vi "TestXYGraph_Buffer_Dbl_VIG.vi"(7 "Operation":T1(ring)=enum."set data", 8 "error in":errorcluster, 9 "XYCluster":cluster{"X":dbl, "Y":dbl}, 10 "index/size":i32, 11 "XY_data_in":cluster{"X":dbl, "Y":dbl}[](array[cluster])) -> (0 "error out":errorcluster, 3 "XY_data_out":cluster{"X":dbl, "Y":dbl}[](array[cluster]))   [LabVIEW 2018]
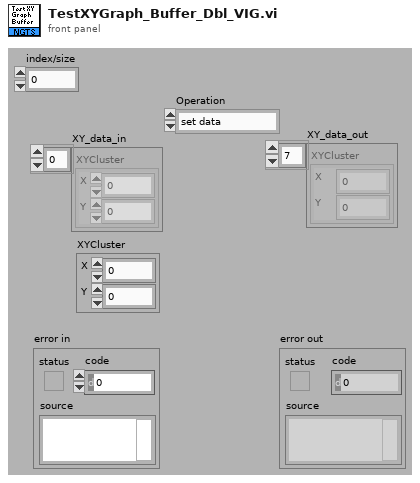
[diagram p1: front panel]
types:
  T1 = enum16{"get data", "set data", "Add Data Pair", "initialize"}
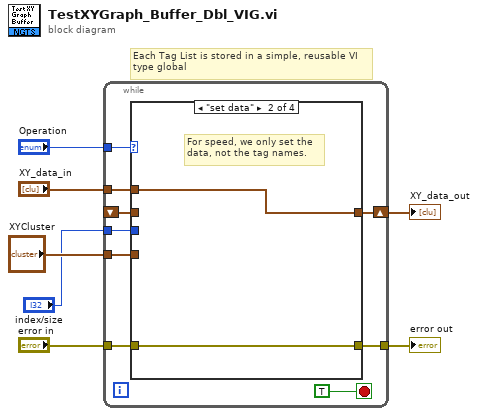
[diagram p0: block diagram]
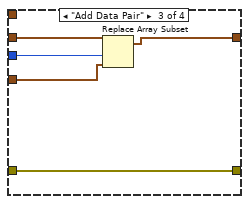
[diagram p3: hidden frame]
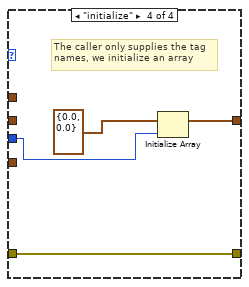
[diagram p4: hidden frame]
diagram:
  # "Each Tag List is stored in a simple, reusable VI\ntype global"
  n1 = while {
    tunnel: "Operation" -> [w16]
    shift-right: [w14] -> w5
    shift-left: _ -> [w12]
    tunnel: "XY_data_in" -> [w13]
    tunnel: "XYCluster" -> [w11]
    tunnel: "error in" -> [w10]
    tunnel: [w9] -> w3
    tunnel: "index/size" -> [w8]
    stop <- TRUE stop-if-true
    n2 = case shown="\"set data\"" w16 {
      tunnel: [w18 w20 w24 w29] -> w14
      tunnel: w13 -> [_ w20 _ _]
      tunnel: w12 -> [w18 _ w25 _]
      tunnel: w11 -> [_ _ w22 _]
      tunnel: w10 -> [w17 w19 w23 w28]
      tunnel: [w17 w19 w23 w28] -> w9
      tunnel: w8 -> [_ _ w21 w26]
      frame "get data", Default {
      }
      frame "set data" {
        # "For speed, we only set the\ndata, not the tag names."
      }
      frame "Add Data Pair" {
        n3 = Replace Array Subset(array=w25, new element=w22, index=w21) -> (w24:cluster{"X":dbl, "Y":dbl}[])
      }
      frame "initialize" {
        # "The caller only supplies the tag\nnames, we initialize an array"
        n4 = Initialize Array(cluster{"X":dbl, "Y":dbl} {"X"=0.0, "Y"=0.0} ("XYCluster"), w26) -> (w29:cluster{"X":dbl, "Y":dbl}[])
      }
    }
  }
  "error out" <- w3
  "XY_data_out" <- w5
